vi "3.1.vi"() -> ()   [LabVIEW 2020]
uses:
  <vilib>/numeric/Random Number (Range) I64.vi
  <vilib>/numeric/sub_Random U32.vi
panel:
  out "Waveform Graph":dbl[][](graph)
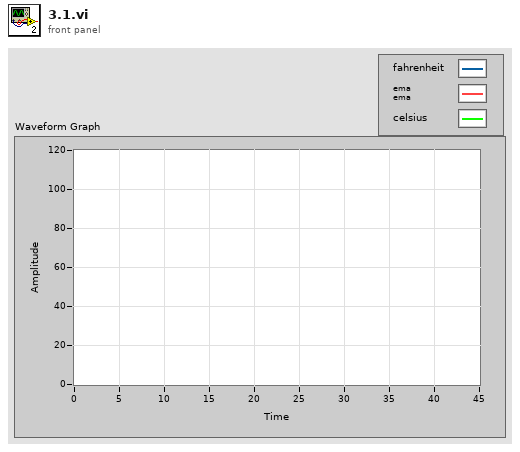
[diagram p1: front panel]
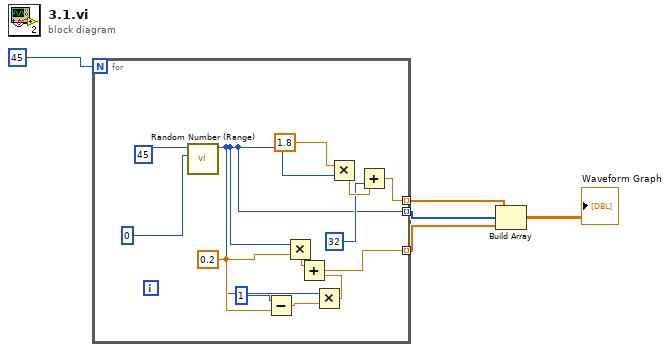
[diagram p0: block diagram]
diagram:
  n1 = for {
    N: 45 -> [_]
    tunnel: [w13] -> w4 mode=indexing
    tunnel: [w6] -> w3 mode=indexing
    tunnel: [w7] -> w2 mode=indexing
    w11 = 0.2
    n2 = call-poly <vilib>:"Random Number (Range).vi"("lower bound (-100)"=0, "upper bound (100)"=45) -> ("number"=w6:i64)  [unwired: 9 in]
    n3 = Subtract(x=1, y=w11) -> (x-y=w8:dbl)
    n4 = Multiply(x=w6, y=w11) -> (x*y=w10:dbl)
    n5 = Multiply(x=w6, y=w8) -> (x*y=w9:dbl)
    n6 = Add(x=w10, y=w9) -> (x+y=w7:dbl)
    n7 = Multiply(x=1.8, y=w6) -> (x*y=w15:dbl)
    n8 = Add(x=w15, y=32) -> (x+y=w13:dbl)
  }
  n9 = Build Array(w4, w3, w2) -> (→"Waveform Graph":dbl[][])
